vi "Angle Calc_Normalize-Accept Beacon Position.vi"(0 "slope":sgl, 5 "Xin":sgl, 7 "Deviation Threshold":sgl format="%#_13g", 9 "intercept":sgl, 11 "Yin":sgl) -> (4 "Accept Beacon":bool, 6 "Xout":sgl, 8 "Distance":sgl, 10 "Perpendicular Slope":sgl format="%#_13g", 15 "Yout":sgl)   [LabVIEW 2015]
panel:
  out "b'":sgl format="%#_13g"
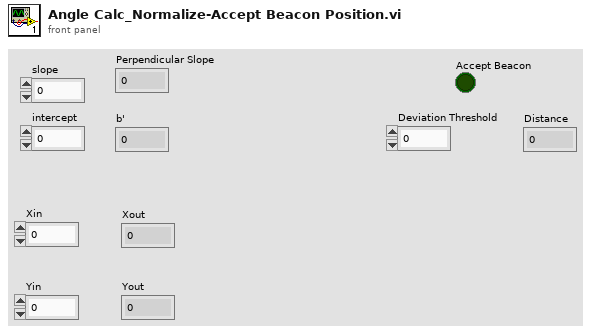
[diagram p1: front panel]
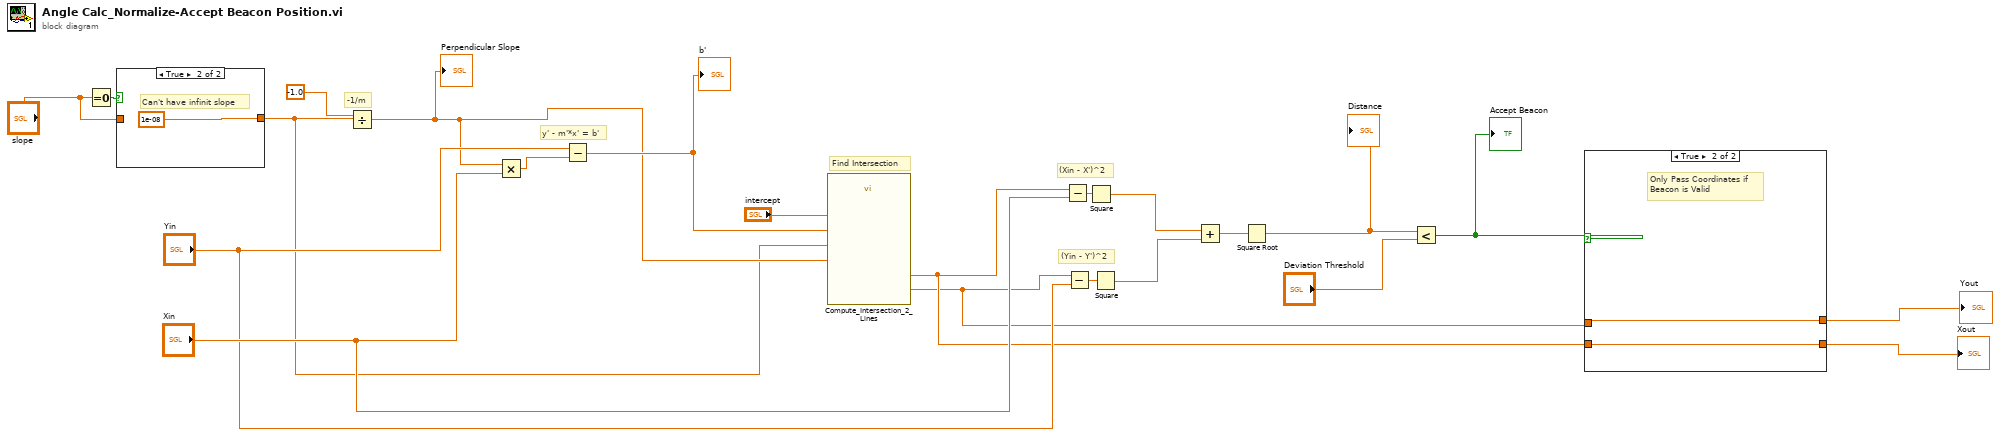
[diagram p0: block diagram]
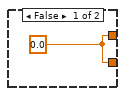
[diagram p3: hidden frame]
diagram:
  # "Find Intersection"
  # "(Yin - Y')^2"
  # "(Xin - X')^2"
  # "-1/m"
  # "y' - m'*x' = b'"
  n1 = Equal To 0?(x="slope") -> (x = 0?=w3:bool)
  n2 = case shown="True" w3 {
    tunnel: [w23 1e-08] -> w2
    tunnel: "slope" -> [w23 _]
    frame False {
    }
    frame True {
      # "Can't have infinit slope"
    }
  }
  n3 = Divide(x=-1.0, y=w2) -> (x/y=w9:dbl)
  "Perpendicular Slope" <- w9
  n4 = Multiply(x=w9, y="Xin") -> (x*y=w21:dbl)
  n5 = Subtract(x="Yin", y=w21) -> (x-y=w20:dbl)
  "b'" <- w20
  n6 = call "Compute_Intersection_2_Lines.vi"("m'"=w9, "b'"=w20, "b"="intercept", "m"=w2) -> ("Yint"=w5:sgl, "Xint"=w8:sgl)  [unwired: 6 in]
  n7 = Subtract(x=w8, y="Xin") -> (x-y=w15:sgl)
  n8 = Subtract(x=w5, y="Yin") -> (x-y=w14:sgl)
  n9 = Square(x=w15) -> (x^2=w13:sgl)
  n10 = Square(x=w14) -> (x^2=w12:sgl)
  n11 = Add(x=w13, y=w12) -> (x+y=w16:sgl)
  n12 = Square Root(x=w16) -> (sqrt(x)=w11:sgl)
  "Distance" <- w11
  n13 = Less?(x=w11, y="Deviation Threshold") -> (x < y?=w4:bool)
  "Accept Beacon" <- w4
  n14 = case shown="True" w4 {
    tunnel: w8 -> [_ w27]
    tunnel: [w25 w27] -> w7
    tunnel: w5 -> [_ w26]
    tunnel: [w25 w26] -> w6
    frame False {
      w25 = 0.0
    }
    frame True {
      # "Only Pass Coordinates if\nBeacon is Valid"
    }
  }
  "Xout" <- w7
  "Yout" <- w6
